vi "Read From Config.vi"(8 "error in (no error)":errorcluster, 11 "DataLogger in":refnum<class "DataLogger.lvclass">) -> (0 "error out":errorcluster, 3 "DataLogger out":refnum<class "DataLogger.lvclass">)   [LabVIEW 2020, in "Volatus.lvlib" / "DataLogger.lvclass"]
uses:
  DataLogger.lvclass
  DataLogger.lvclass/DataLogger.ctl
  Task/Task.lvclass
  VolatusConfig/VolatusConfigElement/VolatusConfigElement.lvclass
  lv-cdm/CDM-Config/Config Element/Config Element.lvclass
  Split Type.ctl
  Volatus.lvlib
  C:/dev/lv20CE/relink/lv-volatus/Volatus/DataHandlerTask/DataHandlerTask.lvclass
  C:/dev/lv20CE/relink/lv-volatus/Volatus/Task/Task.lvclass
  C:/Program Files (x86)/National Instruments/LabVIEW 2020/vi.lib/ActorFramework/Actor/Actor.lvclass
  C:/dev/lv20CE/relink/lv-volatus/Volatus/TaskStateHandler/TaskStateHandler.lvclass
  C:/dev/lv20CE/relink/lv-volatus/Volatus/VectoMessageHandler/VectoMessageHandler.lvclass
  C:/dev/lv20CE/relink/lv-volatus/Volatus/API Provider/API Provider.lvclass
  C:/dev/lv20CE/relink/lv-volatus/Volatus/DataHandler/DataHandler.lvclass
  C:/dev/lv20CE/relink/lv-volatus/Volatus/DataLogger/DataLogger.lvclass
  C:/dev/lv20CE/relink/lv-volatus/Volatus/LoggingHandler/LoggingHandler.lvclass
  VolatusConfig/Task/Task.lvclass
  C:/dev/lv20CE/relink/lv-volatus/VolatusConfig/VolatusConfigElement/VolatusConfigElement.lvclass
  C:/dev/lv20CE/relink/lv-volatus/VolatusConfig/Task/Task.lvclass
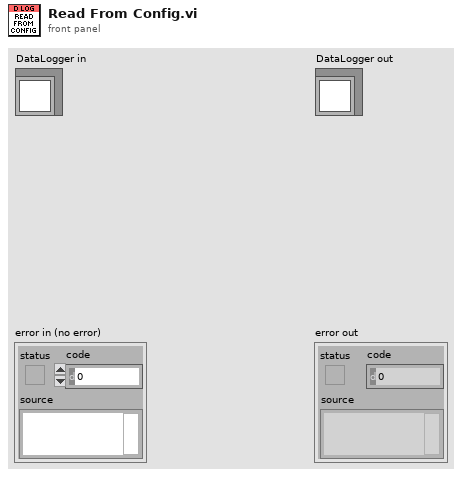
[diagram p1: front panel]
types:
  T1 = typedef "Volatus.lvlib/Split Type.ctl" = enum16{"Count", "Size"}
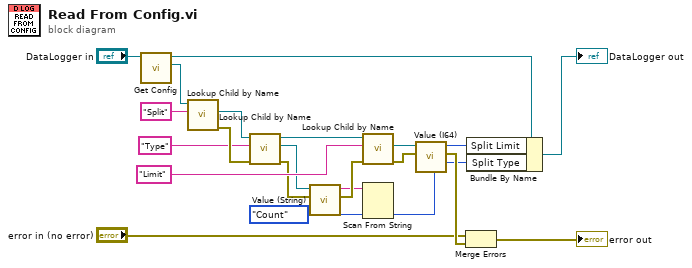
[diagram p0: block diagram]
diagram:
  n1 = call "Get Config.vi"("Task in"="DataLogger in") -> ("Config"=w18:refnum<class "Task.lvclass">, "Task out"=w3:refnum<class "DataLogger.lvclass">)  [unwired: 8 in, 1 out]
  n2 = call "Lookup Child by Name.vi"("Child Name"="Split", "VolatusConfigElement in"=w18) -> ("error out"=w21:errorcluster, "Child"=w16:refnum<class "Config Element.lvclass">)  [unwired: 6 in, 2 out]
  n3 = call "Lookup Child by Name.vi"("error in (no error)"=w21, "Name"="Type" ("Child Name"), "Config Element in"=w16) -> ("error out"=w9:errorcluster, "Child"=w10:refnum<class "Config Element.lvclass">, "Config Element out"=w14:refnum<class "Config Element.lvclass">)  [unwired: 5 in, 1 out]
  n4 = call "Value (String).vi"("error in (no error)"=w9, "Config Element in"=w10) -> ("error out"=w8:errorcluster, "String Value"=w7:string)  [unwired: 8 in]
  n5 = call "Lookup Child by Name.vi"("error in (no error)"=w8, "Name"="Limit" ("Child Name"), "Config Element in"=w14) -> ("error out"=w6:errorcluster, "Child"=w11:refnum<class "Config Element.lvclass">)  [unwired: 5 in, 2 out]
  n6 = Scan From String(input string=w7, default 1=Split_Type."Count" ("Split Type")) -> (output 1=w5:T1)  [unwired: 3 in, 3 out]
  n7 = call "Value (I64).vi"("error in (no error)"=w6, "Config Element in"=w11) -> ("error out"=w22:errorcluster, "I64 Value"=w4:i64)  [unwired: 8 in]
  n8 = Merge Errors("error in (no error)", w22) -> (→"error out":errorcluster)
  n9 = Bundle By Name(cluster=w3, "Split Limit"=w4, "Split Type"=w5) -> (→"DataLogger out":refnum<class "DataLogger.lvclass">)
